vi "Test Assertion Result when Fail.vi"(8 "error in (no error)":errorcluster, 11 "Test Assertion Results in":refnum<class "Assertion Result Test.lvclass">) -> (0 "error out":errorcluster, 3 "Test Assertion Results out":refnum<class "Assertion Result Test.lvclass">)   [LabVIEW 2020, in "LUnit Tests.lvlib" / "Assertion Result Test.lvclass"]
uses:
  Assertion Result Test.lvclass
  C:/Program Files (x86)/National Instruments/LabVIEW 2020/vi.lib/Asteme/LUnit/Test Case.lvclass
  Test Dummys/Test Case Test Double/Test Case Test Double.lvclass
  source/Framework/Result Classes/Assertion Result/Public/TypeDefs/Status.ctl
  <vilib>/Asteme/LUnit/Test Case.lvclass/Test Case.ctl
  <vilib>/Asteme/LUnit/LUnit Assertion Result.lvclass/LUnit Assertion Result.ctl
  <vilib>/Asteme/LUnit/LUnit Test Case Result.lvclass/LUnit Test Case Result.ctl
  <vilib>/Asteme/LUnit/LUnit Method Result.lvclass/LUnit Method Result.ctl
  <vilib>/Asteme/LUnit/Palette/Fail.vi
  <vilib>/Asteme/LUnit/Palette/Pass.vi
  <vilib>/Asteme/LUnit/Set Assertion Type.vi
  <vilib>/Asteme/LUnit/Add test result.vi
  <vilib>/Asteme/LUnit/LUnit Write Passed.vi
  <vilib>/Asteme/LUnit/LUnit Write Message.vi
  <vilib>/Asteme/LUnit/LUnit Write Description.vi
  <vilib>/Asteme/LUnit/LUnit Write Assertion Type.vi
  <vilib>/Asteme/LUnit/LUnit Record Assertion Result.vi
  <vilib>/Asteme/LUnit/LUnit Aggregate Assertion Results.vi
  <vilib>/Asteme/LUnit/Assertion Result/LUnit Read Status.vi
  <vilib>/Asteme/LUnit/LUnit Read Message.vi
  <vilib>/Asteme/LUnit/LUnit Read Description.vi
  <vilib>/Asteme/LUnit/Method Result/LUnit Merge Status.vi
  <vilib>/Asteme/LUnit/LUnit Concatenate result strings.vi
  <vilib>/Asteme/LUnit/LUnit Assertion Result.lvclass
  <vilib>/Asteme/LUnit/Test Case.lvclass
  source/Framework/Result Classes/Assertion Result/Assertion Result.lvclass
  C:/Users/anton/Documents/GitHub/LUnit/tests/Framework Test/Test Assertion Results/Assertion Result Test.lvclass
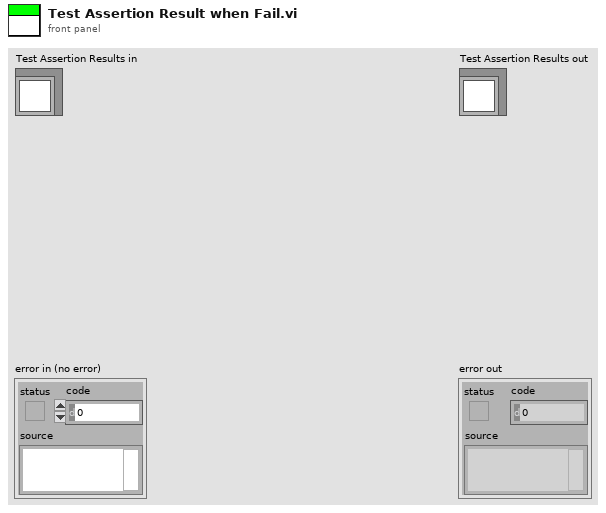
[diagram p1: front panel]
types:
  T1 = typedef "Assertion Result.lvclass/Status.ctl" = enum16{"Pass", "Fail", "Error", "Skipped", "Setup Error", "Broken", "Teardown Error"}
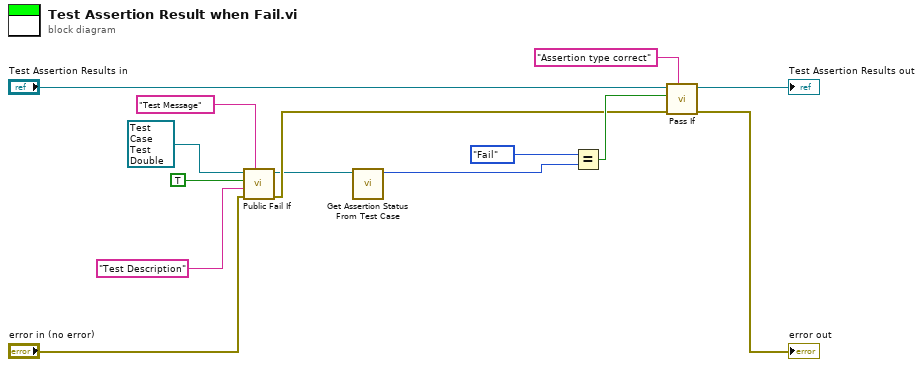
[diagram p0: block diagram]
diagram:
  n1 = call "Public Fail If.vi"("Message"="Test Message", "error in (no error)"="error in (no error)", "Description"="Test Description", "Fail?"=TRUE, "Test Case Test Double in"=refnum<class "Test Case Test Double.lvclass"> refnum ("Test Case Test Double.lvclass")) -> ("error out"=w3:errorcluster, "Test Case Test Double out"=w2:refnum<class "Test Case Test Double.lvclass">)  [unwired: 5 in]
  n2 = call "Get Assertion Status From Test Case.vi"("Test Case Test Double in"=w2) -> ("Status"=w1:T1)  [unwired: 10 in]
  n3 = Equal?(x=Status."Fail", y=w1) -> (x = y?=w7:bool)
  n4 = call <vilib>:"Pass If.vi"("Description"="Assertion type correct", "error in (no error)"=w3, "Pass?"=w7, "LUnit Test Case In"="Test Assertion Results in") -> ("error out"=→"error out":errorcluster, "LUnit Test Case Out"=→"Test Assertion Results out":refnum<class "Assertion Result Test.lvclass">)  [unwired: 6 in]
